vi "write_attributes.vi"(8 "error in (no error)":errorcluster, 10 "attributes":T1, 11 "LassoLarsIC in":refnum<class "LassoLarsIC.lvclass">) -> (0 "error out":errorcluster, 3 "LassoLarsIC out":refnum<class "LassoLarsIC.lvclass">)   [LabVIEW 2020, in "LassoLarsIC.lvclass"]
uses:
  LassoLarsIC.lvclass
  Controls/lasso_lars_ic_attributes.ctl
  LassoLarsIC.lvclass/LassoLarsIC.ctl
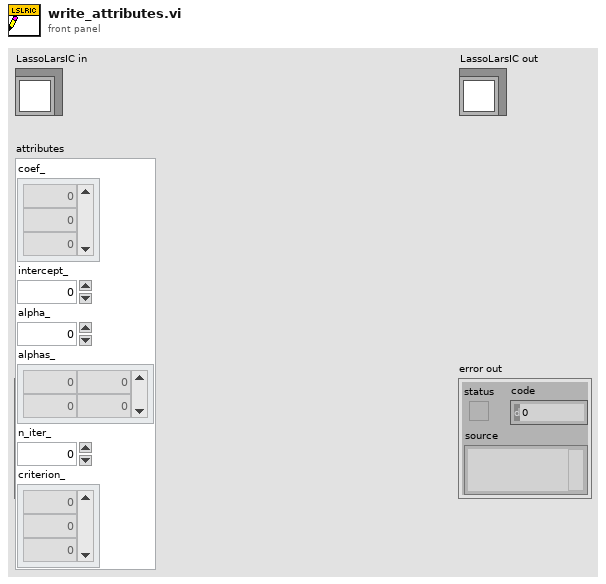
[diagram p1: front panel]
types:
  T1 = typedef "lasso_lars_ic_attributes.ctl" = cluster{"coef_":dbl[], "intercept_":dbl, "alpha_":dbl, "alphas_":dbl[][], "n_iter_":dbl, "criterion_":dbl[]}
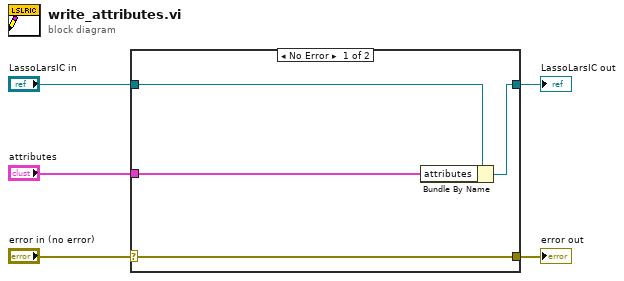
[diagram p0: block diagram]
diagram:
  n1 = case shown="No Error" "error in (no error)" {
    selector: "error in (no error)" -> [w9 w10]
    tunnel: [w9 w10] -> w4
    tunnel: [w7 w11] -> w2
    tunnel: "LassoLarsIC in" -> [w8 w11]
    tunnel: "attributes" -> [w6 _]
    frame No Error {
      n2 = Bundle By Name(cluster=w8, "attributes"=w6) -> (w7:refnum<class "LassoLarsIC.lvclass">)
    }
    frame Error {
    }
  }
  "error out" <- w4
  "LassoLarsIC out" <- w2
